vi "GetPoint.vi"(8 "error in (no error)":errorcluster, 11 "Picture2D in":refnum<class "Picture2D.lvclass">) -> (0 "error out":errorcluster, 2 "Point":refnum<class "Point.lvclass">, 3 "Picture2D out":refnum<class "Picture2D.lvclass">)   [LabVIEW 2021, in "Picture2D.lvlib" / "Picture2D.lvclass"]
uses:
  Picture2D.lvclass
  Point/Point.lvclass
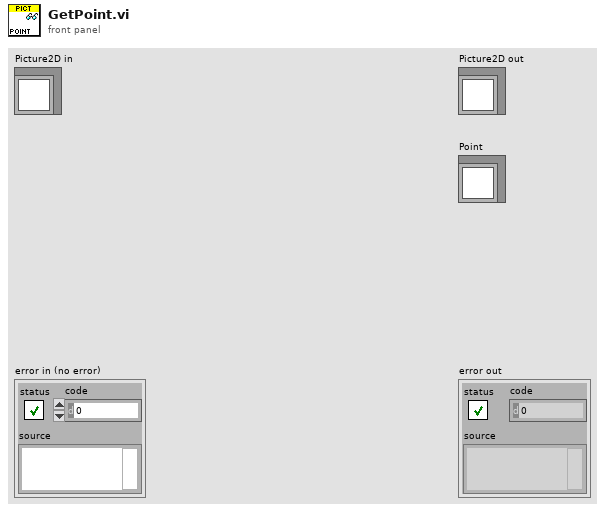
[diagram p1: front panel]
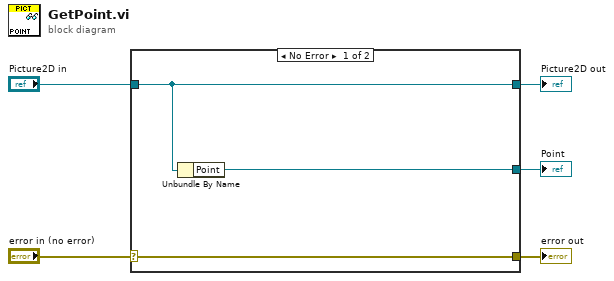
[diagram p0: block diagram]
diagram:
  n1 = case shown="No Error" "error in (no error)" {
    selector: "error in (no error)" -> [w8 w9]
    tunnel: [w8 w9] -> w4
    tunnel: [w7 w10] -> w2
    tunnel: "Picture2D in" -> [w7 w10]
    tunnel: [w6 _] -> w1
    frame No Error {
      n2 = Unbundle By Name(w7) -> ("Point"=w6:refnum<class "Point.lvclass">)
    }
    frame Error {
    }
  }
  "error out" <- w4
  "Picture2D out" <- w2
  "Point" <- w1
